vi "Create Methods List.vi"(8 "error in (no error)":errorcluster, 11 "Methods ListCtrl":refnum<vi>) -> (0 "error out":errorcluster, 3 "Methods ListCtrl 2":refnum<vi>)   [LabVIEW 2017, in "WebServiceImporter.lvlib" / "Main Panel.lvlib" / "Select Methods.lvlib"]
uses:
  <vilib>/Platform/WebService/Main Panel/Pages/Select Methods/Select Methods.lvlib
  <vilib>/Platform/WebService/ProxyDll Generator/ProxyDll Generator.lvlib
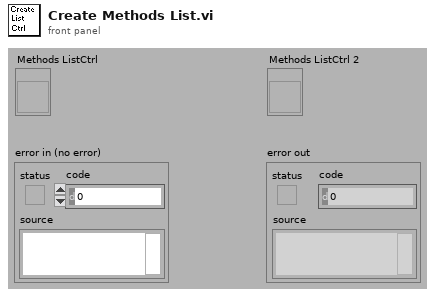
[diagram p1: front panel]
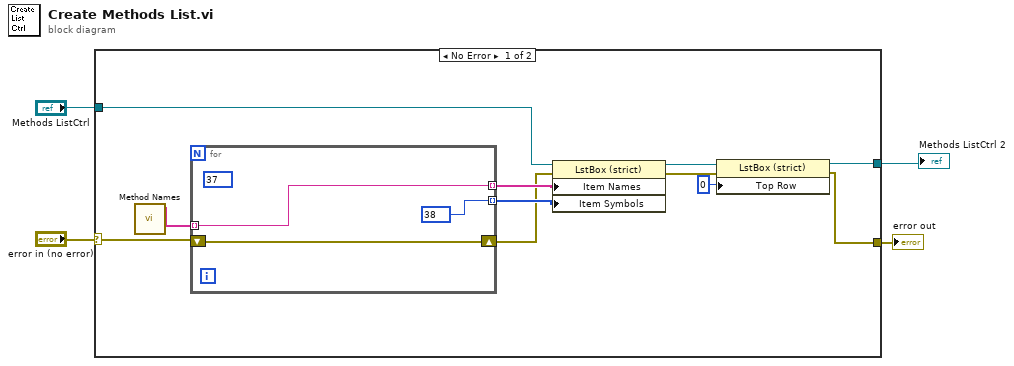
[diagram p0: block diagram]
diagram:
  n1 = case shown="No Error" "error in (no error)" {
    selector: "error in (no error)" -> [w11 w20]
    tunnel: "Methods ListCtrl" -> [w10 w19]
    tunnel: [w6 w20] -> w3
    tunnel: [w5 w19] -> w1
    frame No Error {
      n2 = call <vilib>:"Method Names.vi"() -> ("Method Names (out)"=w12:string[])  [unwired: 10 in, 1 out]
      n3 = for {
        shift-right: [w18] -> w13
        shift-left: w11 -> [w18]
        tunnel: w12 -> [w17] mode=indexing
        tunnel: [w17] -> w15 mode=indexing
        tunnel: [38] -> w14 mode=indexing
        (unwired) 37
      }
      n4 = property class="LstBox (strict)"(reference=w10, error in=w13, "Item Names"=w15, "Item Symbols"=w14) -> (reference out=w9:refnum<vi>, error out=w8:errorcluster)
      n5 = property class="LstBox (strict)"(reference=w9, error in=w8, "Top Row"=0 ("Value")) -> (reference out=w5:refnum<vi>, error out=w6:errorcluster)
    }
    frame Error {
    }
  }
  "error out" <- w3
  "Methods ListCtrl 2" <- w1
